vi "Temperature1(Post).vi"(7 "LabVIEW Web Service Request":refnum<class "Web Request.lvclass">) -> ()   [LabVIEW 2019]
uses:
  <vilib>/wsapi/Web Request.lvclass
  QDMH support files/QDMH Poly VIs/QDMH POLY Enqueue Cluster.vi
panel:
  # "Use the Web Service Request input terminal to call the VIs on the Web Services palette. Do not remove it from the connector pane unless you don't need access to the palette."
  # "Each additional control wired to the connector pane will be available as an input in the URL. To include an indicator in terminal-mode output (the default setting), it must also be wired to the connector pane."
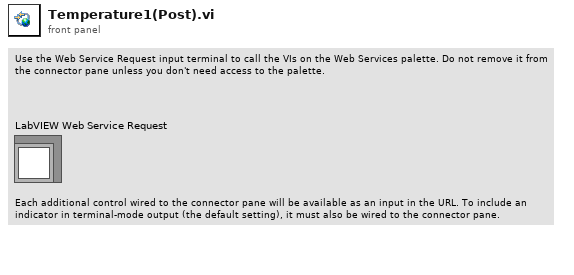
[diagram p1: front panel]
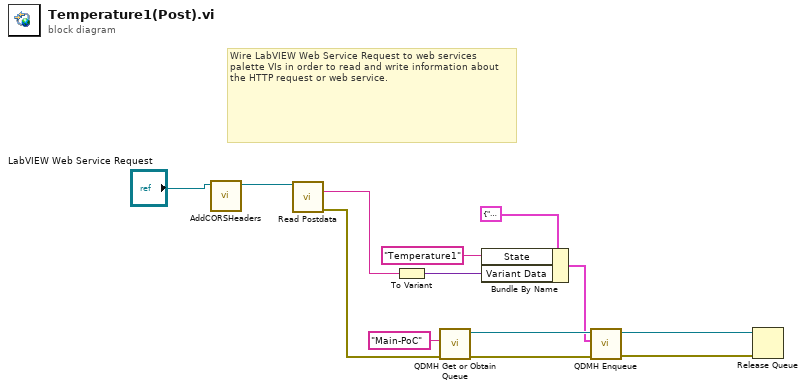
[diagram p0: block diagram]
diagram:
  # "Wire LabVIEW Web Service Request to web services palette VIs in order to read and write information about the HTTP request or web service."
  n1 = call "AddCORSHeaders.vi"("Web Request in"="LabVIEW Web Service Request") -> ("Web Request out"=w13:refnum<class "Web Request.lvclass">)  [unwired: 10 in]
  n2 = call <vilib>:"Read Postdata.vi"("LabVIEW Web Service Request"=w13) -> ("postdata"=w5:string, "error out"=w8:errorcluster)  [unwired: 12 in, 1 out]
  n3 = To Variant(anything=w5) -> (Variant=w4:variant)
  n4 = call "QDMH Get or Obtain Queue.vi"("error in (no error)"=w8, "Queue Name"="Main-PoC") -> ("error out"=w9:errorcluster, "queue out"=w10:refnum<queue>)  [unwired: 1 in, 7 out]
  n5 = Bundle By Name(cluster=cluster{"State":string, "Variant Data":variant} {"State"="", "Variant Data"=variant} ("QDSM Element"), "State"="Temperature1", "Variant Data"=w4) -> (w3:cluster{"State":string, "Variant Data":variant})
  n6 = call-poly "QDMH Enqueue.vi"("error in (no error)"=w9, "QDSM Element"=w3, "queue"=w10) -> ("error out"=w1:errorcluster, "queue out"=w2:refnum<queue>)  [unwired: 7 out]
  n7 = Release Queue(queue=w2, error in (no error)=w1) -> ()  [unwired: 1 in, 3 out]
